vi "Connect PV.vi"(8 "error in (no error)":errorcluster, 10 "PV URL":string, 11 "CS++DIMMonitor in":refnum<class "CS++DIMMonitor.lvclass">) -> (0 "error out":errorcluster, 3 "CS++DIMMonitor out":refnum<class "CS++DIMMonitor.lvclass">)   [LabVIEW 2014, in "CS++DIMMonitor.lvlib" / "CS++DIMMonitor.lvclass"]
doc: "Open connection to process variable."
uses:
  CS++DIMMonitor.lvclass
  DimLVEvent/LVDimInterface/LVDimInterface.lvlib
  DimLVEvent/LVDimInterface/LVDimInterface.dic_info_service_queue.vi
  DimLVEvent/LVDimInterface/LVDimInterface.dim service type.ctl
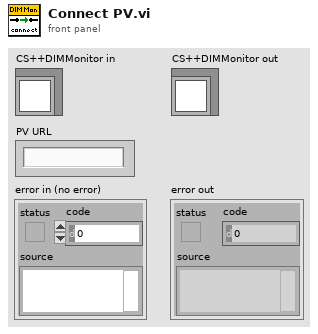
[diagram p1: front panel]
types:
  T1 = typedef "LVDimInterface.lvlib/LVDimInterface.dim service type.ctl" = u16
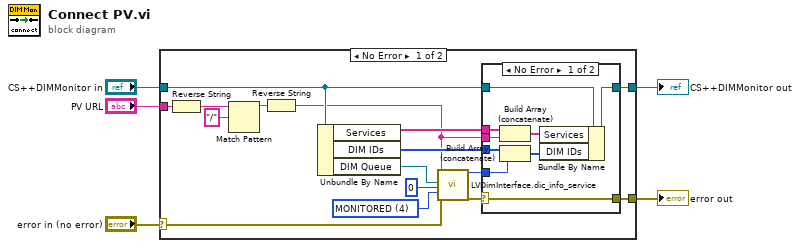
[diagram p0: block diagram]
diagram:
  n1 = case shown="No Error" "error in (no error)" {
    selector: "error in (no error)" -> [w6 w33]
    tunnel: "PV URL" -> [w15 _]
    tunnel: "CS++DIMMonitor in" -> [w14 w34]
    tunnel: [w13 w34] -> w3
    tunnel: [w7 w33] -> w2
    frame No Error {
      w20 = T1 4 items=["ONCE_ONLY"=1, "TIMED"=2, "MONITORED"=4] ("serviceType")
      n2 = Reverse String(1:w15) -> (0:w17:string)
      n3 = Match Pattern(string=w17, regular expression="/" ("search string/char (-)")) -> (before substring=w16:string)  [unwired: 1 in, 3 out]
      n4 = Reverse String(1:w16) -> (0:w9:string)
      n5 = Unbundle By Name(w14) -> ("Services"=w10:string[], "DIM IDs"=w12:i32[], "DIM Queue"=w19:refnum<queue>)
      n6 = call-poly "LVDimInterface.dic_info_service.vi"("serviceName"=w9, "queueRef"=w19, "timeout [s]"=0, "serviceType"=w20, "error in (no error)"=w6) -> ("callBackID"=w11:i32, "error out"=w8:errorcluster)  [unwired: 13 in]
      n7 = case shown="No Error" w8 {
        selector: w8 -> [w22 w31]
        tunnel: w14 -> [w30 w32]
        tunnel: [w29 w32] -> w13
        tunnel: w12 -> [w28 _]
        tunnel: w11 -> [w27 _]
        tunnel: w10 -> [w25 _]
        tunnel: w9 -> [w24 _]
        tunnel: [w22 w31] -> w7
        frame No Error {
          n8 = Build Array (concatenate)(w25, w24) -> (w23:string[])
          n9 = Build Array (concatenate)(w28, w27) -> (w26:i32[])
          n10 = Bundle By Name(cluster=w30, "Services"=w23, "DIM IDs"=w26) -> (w29:refnum<class "CS++DIMMonitor.lvclass">)
        }
        frame Error {
        }
      }
    }
    frame Error {
    }
  }
  "error out" <- w2
  "CS++DIMMonitor out" <- w3
